vi "IScanMoveXYZ.vi"(3 "ZPos":dbl, 4 "YPos":dbl, 5 "XPos":dbl, 6 "PRIORLib.IScanIn":refnum<k7>) -> (0 "Return":i32, 1 "error out":errorcluster, 2 "PRIORLib.IScanOut":refnum<k7>)   [LabVIEW 2011]
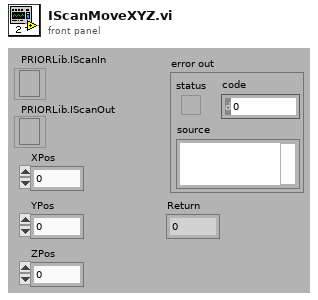
[diagram p1: front panel]
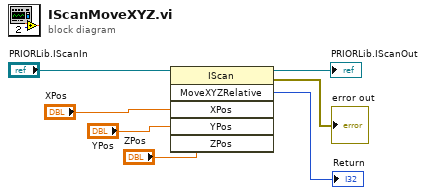
[diagram p0: block diagram]
diagram:
  n1 = invoke class="IScan" method="MoveXYZRelative"(reference="PRIORLib.IScanIn", "XPos"="XPos", "YPos"="YPos", "ZPos"="ZPos") -> (reference out=→"PRIORLib.IScanOut":refnum<k7>, error out=→"error out":errorcluster, "MoveXYZRelative"=→"Return":i32)  [unwired: 2 in, 3 out]
